vi "Excel Merge Cells.vi"(0 "report in":refnum<class "NI_report.lvclass">, 7 "start (-1, -1)":cluster{"row":i32, "column":i32}={"row"=-1, "column"=-1}, 9 "end (-1, -1)":cluster{"row":i32, "column":i32}={"row"=-1, "column"=-1}, 11 "error in (no error)":errorcluster, 12 "name (\"\")":string) -> (4 "report out":refnum<class "NI_report.lvclass">, 15 "error out":errorcluster)   [LabVIEW 2016, in "NI_Excel.lvclass"]
doc: "Merges the range of cells specified by the <B>start</B> and <B>end</B> clusters."
uses:
  <vilib>/Utility/NIReport.llb/Excel/NI_Excel.lvclass
  <vilib>/Utility/NIReport.llb/NI_report.lvclass
  C:/Program Files (x86)/National Instruments/LabVIEW 2016/vi.lib/Utility/NIReport.llb/NI_report.lvclass
  <vilib>/Utility/NIReport.llb/Excel/NI_Excel.lvclass/NI_Excel.ctl
  <vilib>/addons/_office/NI_ReportGenerationToolkit.lvlib
  <vilib>/Utility/NIReport.llb/NI_ReportGenerationCore.lvlib
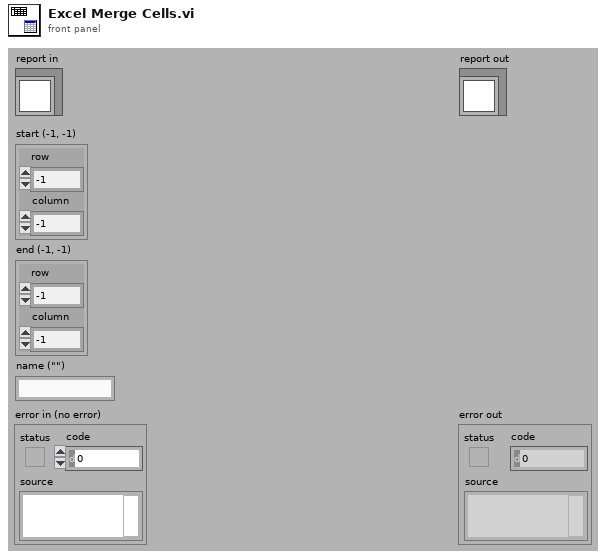
[diagram p1: front panel]
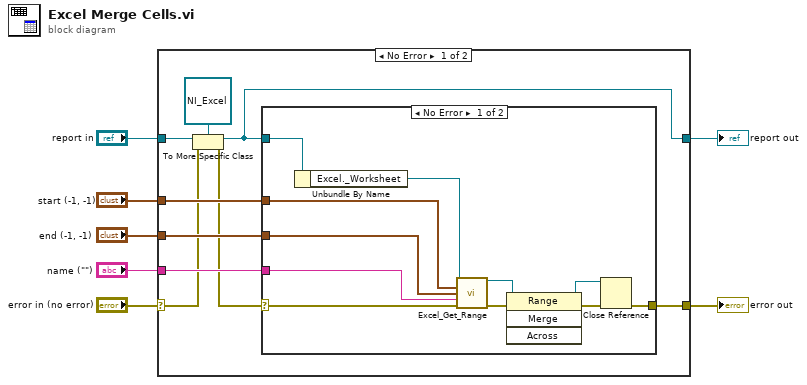
[diagram p0: block diagram]
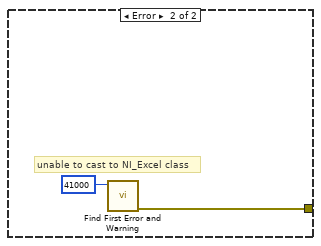
[diagram p2: hidden frame]
diagram:
  n1 = case shown="No Error" "error in (no error)" {
    selector: "error in (no error)" -> [w8 w31]
    tunnel: [w16 w31] -> w6
    tunnel: [w10 w30] -> w4
    tunnel: "report in" -> [w11 w30]
    tunnel: "start (-1, -1)" -> [w15 _]
    tunnel: "end (-1, -1)" -> [w14 _]
    tunnel: "name (\"\")" -> [w13 _]
    frame No Error {
      n2 = To More Specific Class(target class=refnum<class "NI_Excel.lvclass"> refnum ("report in"), reference=w11, error in=w8) -> (specific class reference=w10:refnum<class "NI_Excel.lvclass">, error out=w9:errorcluster)
      n3 = case shown="No Error" w9 {
        selector: w9 -> [w17 _]
        tunnel: [w24 w28] -> w16
        tunnel: w15 -> [w22 _]
        tunnel: w14 -> [w21 _]
        tunnel: w13 -> [w20 _]
        tunnel: w10 -> [w18 _]
        frame No Error {
          n4 = Unbundle By Name(w18) -> ("Excel._Worksheet"=w23:refnum<k7>)
          n5 = call <vilib>:"Excel_Get_Range.vi"("Excel._Worksheet"=w23, "start"=w22, "end"=w21, "name"=w20, "error in (no error)"=w17) -> ("Range"=w19:refnum<k7>, "error out"=w27:errorcluster)  [unwired: 5 in, 4 out]
          n6 = invoke class="Range" method="Merge"(reference=w19, error in=w27) -> (reference out=w26:refnum<k7>, error out=w25:errorcluster)  [unwired: 2 in, 2 out]
          n7 = Close Reference(reference=w26, error in (no error)=w25) -> (error out=w24:errorcluster)
        }
        frame Error {
          # "unable to cast to NI_Excel class"
          n8 = call <vilib>:"Find First Error and Warning.vi"("error code"=41000) -> ("error out"=w28:errorcluster)  [unwired: 2 in, 4 out]
        }
      }
    }
    frame Error {
    }
  }
  "error out" <- w6
  "report out" <- w4
